vi "Calibration(XY).vi"(7 "Load calibration data":bool, 8 "error in (no error)":errorcluster, 9 "Save calibration data":bool, 10 "Done Button":bool, 11 "Acceleration [g]| Voltage [V]":dbl[][](array[numeric])=[[3.0, 3.3], [0.0, 1.64], [-3.0, 0.25], [1.0, 1.95]]) -> (0 "error out":errorcluster, 2 "Interpolation method":T1(ring), 3 "Distance [cm]| Voltage [V]":dbl[][](array[numeric])=[[3.0, 3.3], [0.0, 1.64], [-3.0, 0.25], [1.0, 1.95]])   [LabVIEW 2025]
uses:
  <vilib>/Utility/file.llb/Write To Spreadsheet File (DBL).vi
  <vilib>/Utility/file.llb/Read From Spreadsheet File (DBL).vi
  <vilib>/gmath/NI_Gmath.lvlib
panel:
  in  "method":T1(ring)=enum."linear"
  in  "Refresh Button":bool
  out "Transfer function":cluster{"yi":dbl[], "xi used":dbl[]}[](graph)=[{"yi"=[3.3, 1.64, 0.25, 1.95], "xi used"=[3.0, 0.0, -3.0, 1.0]}, {"yi"=[0.25, 0.2934375, 0.336875, 0.38031249999999994, 0.42374999999999996, 0.4671874999999999, 0.5106249999999999, 0.5540624999999999, 0.5974999999999999, 0.6409374999999999, 0.684375, 0.7278125, 0.77125, 0.8146875, 0.858125, 0.9015625, 0.945, 0.9884374999999999, 1.0318749999999999, 1.0753125, 1.11875, 1.1621875, 1.205625, 1.2490625, 1.2925, 1.3359375, 1.379375, 1.4228125, 1.46625, 1.5096875, 1.553125, 1.5965625, 1.64, 1.6496874999999998, 1.6593749999999998, 1.6690625, 1.67875, 1.6884375, 1.6981249999999999, 1.7078124999999997, 1.7174999999999998, 1.7271874999999999, 1.736875, 1.7465625, 1.7562499999999999, 1.7659374999999997, 1.7756249999999998, 1.7853124999999999, 1.795, 1.8046875, 1.814375, 1.8240625000000001, 1.83375, 1.8434374999999998, 1.853125, 1.8628125, 1.8725, 1.8821875000000001, 1.891875, 1.9015624999999998, 1.91125, 1.9209375, 1.930625, 1.9403125, 1.95, 1.9921875, 2.034375, 2.0765624999999996, 2.11875, 2.1609375, 2.203125, 2.2453125, 2.2875, 2.3296875000000004, 2.371875, 2.4140625, 2.45625, 2.4984374999999996, 2.540625, 2.5828125, 2.625, 2.6671875, 2.709375, 2.7515625000000004, 2.79375, 2.8359375, 2.878125, 2.9203124999999996, 2.9625, 3.0046875, 3.046875, 3.0890625, 3.1312499999999996, 3.1734374999999995, 3.2156249999999997, 3.2578125, 3.3], "xi used"=[-3.0, -2.90625, -2.8125, -2.71875, -2.625, -2.53125, -2.4375, -2.34375, -2.25, -2.15625, -2.0625, -1.96875, -1.875, -1.78125, -1.6874999999999998, -1.5937499999999998, -1.5, -1.40625, -1.3125, -1.21875, -1.125, -1.03125, -0.9375, -0.84375, -0.75, -0.6562499999999999, -0.5624999999999998, -0.4687499999999997, -0.37499999999999967, -0.28124999999999956, -0.1874999999999995, -0.09374999999999942, 0.0, 0.03124999999999939, 0.06249999999999967, 0.09374999999999994, 0.12500000000000022, 0.1562500000000005, 0.1874999999999999, 0.21874999999999928, 0.24999999999999956, 0.28124999999999983, 0.3125000000000001, 0.3437500000000004, 0.3749999999999998, 0.40624999999999917, 0.43749999999999944, 0.4687499999999997, 0.5, 0.5312500000000002, 0.5625000000000006, 0.5937500000000009, 0.6250000000000002, 0.6562499999999996, 0.6874999999999999, 0.7187500000000002, 0.7500000000000004, 0.7812500000000007, 0.8125000000000001, 0.8437499999999996, 0.8749999999999998, 0.90625, 0.9375000000000003, 0.9687500000000007, 1.0, 1.0625, 1.125, 1.1875, 1.25, 1.3125, 1.375, 1.4375, 1.5, 1.5625, 1.625, 1.6875, 1.75, 1.8125, 1.875, 1.9375, 2.0, 2.0625, 2.125, 2.1875, 2.25, 2.3125, 2.375, 2.4375, 2.5, 2.5625, 2.625, 2.6875, 2.75, 2.8125, 2.875, 2.9375, 3.0]}]
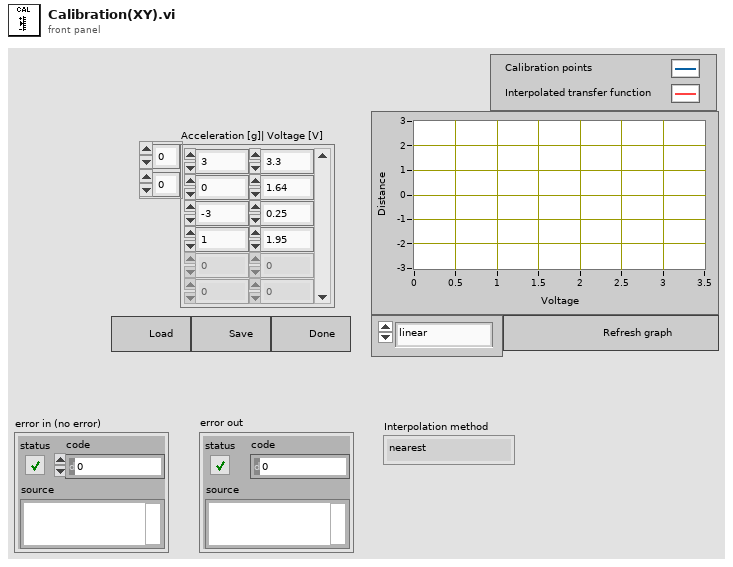
[diagram p1: front panel]
types:
  T1 = enum16{"nearest", "linear", "spline", "cubic Hermite", "Lagrange"}
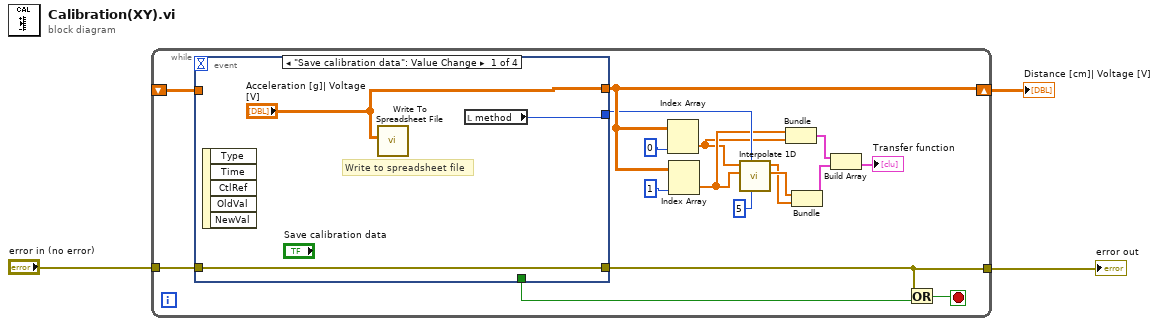
[diagram p0: block diagram]
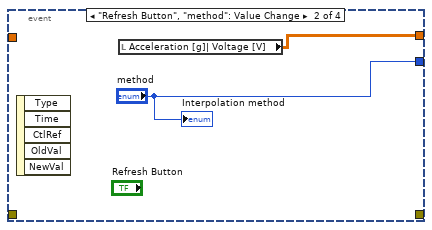
[diagram p2: hidden frame]
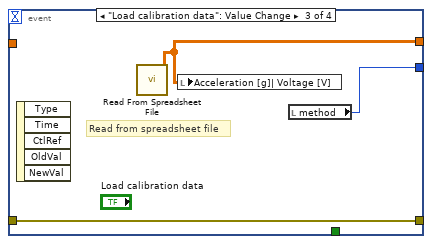
[diagram p3: hidden frame]
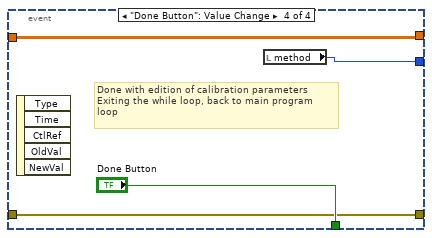
[diagram p4: hidden frame]
diagram:
  n1 = while {
    tunnel: "error in (no error)" -> [w19]
    tunnel: [w18] -> w3
    shift-right: [w13] -> w1
    shift-left: _ -> [w20]
    stop <- w16 stop-if-true
    n2 = event shown="[0] \"Save calibration data\": Value Change" {
      selector: _ -> [_ _ _ _]
      dyn-events: _ -> [_ _ _ _]
      timeout: _ -> [_ _ _ _]
      tunnel: w20 -> [_ _ _ w32]
      tunnel: ["Acceleration [g]| Voltage [V]" w25 w27 w32] -> w13
      tunnel: [_ _ _ "Done Button"] -> w17
      tunnel: w19 -> [w23 _ w28 w30]
      tunnel: [w23 _ w28 w30] -> w18
      tunnel: [w21 "method" w26 w29] -> w8
      event "Save calibration data": Value Change {
        # "Write to spreadsheet file"
        n3 = event-data() -> ()  [unwired: 1 in, 5 out]
        n4 = call-poly <vilib>:"Write To Spreadsheet File.vi"("2D data"="Acceleration [g]| Voltage [V]") -> ()  [unwired: 7 in, 1 out]
        n5 = local read "method"() -> (w21:T1)
      }
      event "Refresh Button", "method": Value Change {
        n6 = event-data() -> ()  [unwired: 1 in, 5 out]
        n7 = local read "Acceleration [g]| Voltage [V]"() -> (w25:dbl[][])
        "Interpolation method" <- "method"
      }
      event "Load calibration data": Value Change {
        # "Read from spreadsheet file"
        n8 = event-data() -> ()  [unwired: 1 in, 5 out]
        n9 = call-poly <vilib>:"Read From Spreadsheet File.vi"() -> ("all rows"=w27:dbl[][])  [unwired: 7 in, 4 out]
        n10 = local write "Acceleration [g]| Voltage [V]"(w27) -> ()
        n11 = local read "method"() -> (w26:T1)
      }
      event "Done Button": Value Change {
        # "Done with edition of calibration parameters\nExiting the while loop, back to main program \nloop"
        n12 = event-data() -> ()  [unwired: 1 in, 5 out]
        n13 = local read "method"() -> (w29:T1)
      }
    }
    n14 = Index Array(array=w13, index (col)=0 ("disabled index (col)")) -> (element=w6:dbl[])  [unwired: 1 in]
    n15 = Index Array(array=w13, index (col)=1 ("disabled index (col)")) -> (element=w7:dbl[])  [unwired: 1 in]
    n16 = call <vilib>:"Interpolate 1D.vi"("ntimes"=5, "method"=w8, "X"=w7, "Y"=w6) -> ("xi used"=w5:dbl[], "yi"=w4:dbl[])  [unwired: 5 in, 1 out]
    n17 = Bundle("all rows"=w7, "all rows"=w6) -> (w11:cluster{"all rows":dbl[], "all rows":dbl[]})  [unwired: 1 in]
    n18 = Bundle("xi used"=w5, "yi"=w4) -> (w10:cluster{"xi used":dbl[], "yi":dbl[]})  [unwired: 1 in]
    n19 = Build Array(w11, w10) -> (→"Transfer function":cluster{"xi used":dbl[], "yi":dbl[]}[])
    n20 = Or(x=w18, y=w17) -> (x .or. y?=w16:bool)
  }
  "error out" <- w3
  "Distance [cm]| Voltage [V]" <- w1
